vi "DidInit.vi"(7 "Init?":bool, 8 "error in (no error)":errorcluster, 11 "ModuleAdmin":refnum<class "ModuleAdmin.lvclass">) -> (0 "error out":errorcluster)   [LabVIEW 2018, in "AcPwrPlugins.lvlib"]
doc: "This VI broadcasts that Main.vi has been initialized."
uses:
  AcPwrPlugins.lvlib
  <userlib>/NIST/ModuleAdminLib/ModuleAdmin/ModuleAdmin.lvclass
  AcPwrShared/clEventType.ctl
  AcPwrShared/clDidInit.ctl
  AcPwrShared/AcPwrShared.lvlib
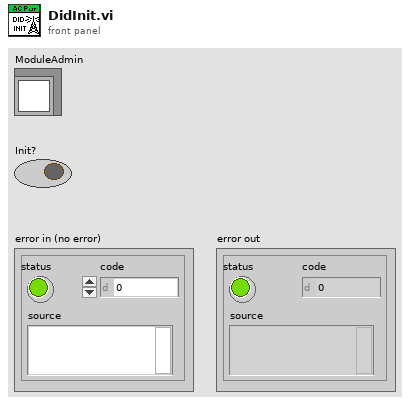
[diagram p1: front panel]
types:
  T1 = typedef "AcPwrShared.lvlib/clDidInit.ctl" = cluster{"Init?":bool, "ModuleAdmin":refnum<class "ModuleAdmin.lvclass">}
  T2 = typedef "AcPwrShared.lvlib/clEventType.ctl" = cluster{"ModuleID":i32, "Data":variant}
  T3 = typedef "AcPwrShared.lvlib/clBroadcastEvents.ctl" = cluster{"DidInit":refnum<user-event>, "StatusUpdate":refnum<user-event>, "ErrorReport":refnum<user-event>, "DidStop":refnum<user-event>, "PathToINI":refnum<user-event>, "Measurements":refnum<user-event>, "LoadConfigFile":refnum<user-event>, "GetSettings":refnum<user-event>, "SetSettings":refnum<user-event>, "GetType&ID":refnum<user-event>, "GotSettings":refnum<user-event>}
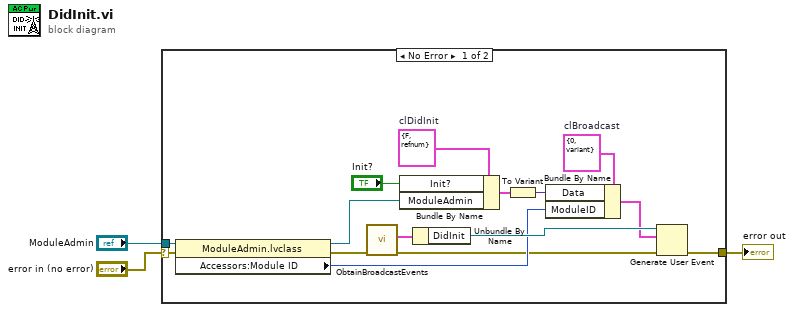
[diagram p0: block diagram]
diagram:
  n1 = case shown="No Error" "error in (no error)" {
    selector: "error in (no error)" -> [w7 w19]
    tunnel: [w11 w19] -> w3
    tunnel: "ModuleAdmin" -> [w9 _]
    frame No Error {
      w18 = T1 {"Init?"=FALSE, "ModuleAdmin"=refnum}  # clDidInit
      w14 = T2 {"ModuleID"=0, "Data"=variant}  # clBroadcast
      n2 = property class="ModuleAdmin.lvclass"(reference=w9, error in=w7) -> (reference out=w6:refnum<class "ModuleAdmin.lvclass">, error out=w5:errorcluster, "Accessors:Module ID"=w8:i32)
      n3 = call "ObtainBroadcastEvents.vi"("error in (no error)"=w5) -> ("error out"=w4:errorcluster, "clAcPwrEvents"=w17:T3)  [unwired: 9 in]
      n4 = Bundle By Name(cluster=w18, "Init?"="Init?", "ModuleAdmin"=w6) -> (w16:T1)
      n5 = Unbundle By Name(w17) -> ("DidInit"=w15:refnum<user-event>)
      n6 = To Variant(anything=w16) -> (Variant=w13:variant)
      n7 = Bundle By Name(cluster=w14, "Data"=w13, "ModuleID"=w8) -> (w12:T2)
      n8 = Generate User Event(user event=w15, event data cluster=w12, error in=w4) -> (error out=w11:errorcluster)  [unwired: 1 in, 1 out]
    }
    frame Error {
    }
  }
  "error out" <- w3
